vi "Previous Station Check.vi"() -> ()   [LabVIEW 2015]
uses:
  Control Button/rpt.ctl
  <vilib>/Utility/error.llb/whitespace.ctl
  <vilib>/addons/database/Connection.llb/DB Tools Open Connec (String).vi
  Galobal variable_TI.vi
  <vilib>/Utility/file.llb/Read Delimited Spreadsheet (string).vi
  Project Setup/Globle Variable/GR_Servo.vi
  <vilib>/Utility/file.llb/Write Delimited Spreadsheet (string).vi
  <vilib>/addons/database/NI_Database_API.lvlib
panel:
  out "error out 5":errorcluster
  out "array 2":string[][](array[string])
  out "error out 4":errorcluster
  out "size(s)":i32
  out "error out 3":errorcluster
  out "array":string[][](array[string])
  out "error out 2":errorcluster
  out "error out":errorcluster
  in  "stop":bool
  in  "RPT":T1
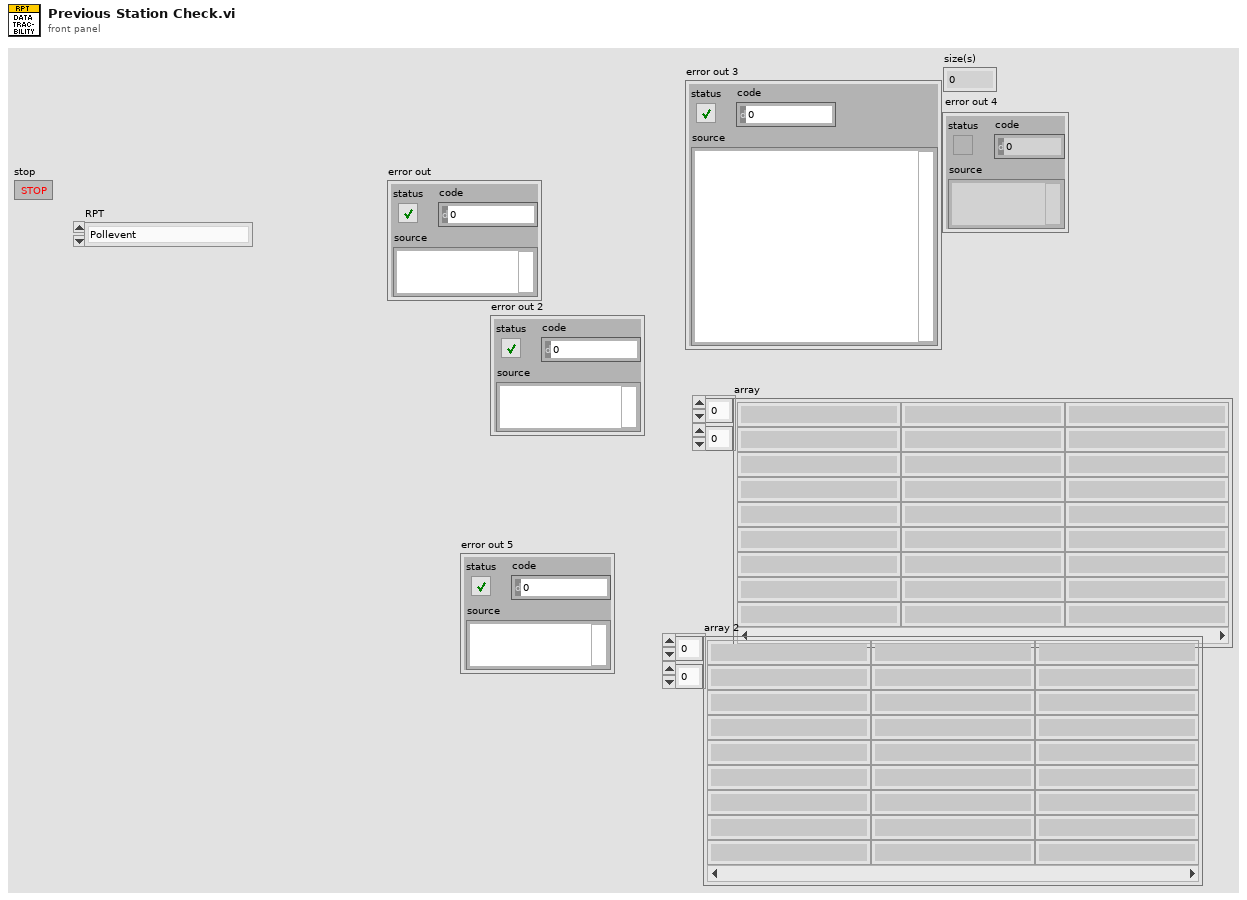
[diagram p1: front panel]
types:
  T1 = typedef "rpt.ctl" = enum16{"Pollevent", "Read", "Write", "Delete"}
  T2 = cluster{"Stn Name":string, "date":string, "time":string, "Operator id":string, "Shift":string, "Error Code":string, "Fail count":string, "Rework":string, "NA":string, "Tested":string}
  T3 = typedef "NI_Database_API.lvlib/Conn ObjectReference.ctl" = refnum<k1>
  T4 = enum16{"open", "replace", "create", "open or create", "replace or create", "replace or create with confirmation"}
  T5 = typedef "whitespace.ctl" = u16
  T6 = cluster{"Report data[0]":string, "Report data[1]":string, "Report data[2]":string, "Report data[3]":string, "Report data[4]":string, "Report data[5]":string, "Report data[6]":string, "Report data[7]":string, "Report data[8]":string, "Report data[9]":string, "Report data[10]":string, "Report data[11]":string, "Report data[12]":string, "Report data[13]":string, "Report data[14]":string, "Report data[15]":string}
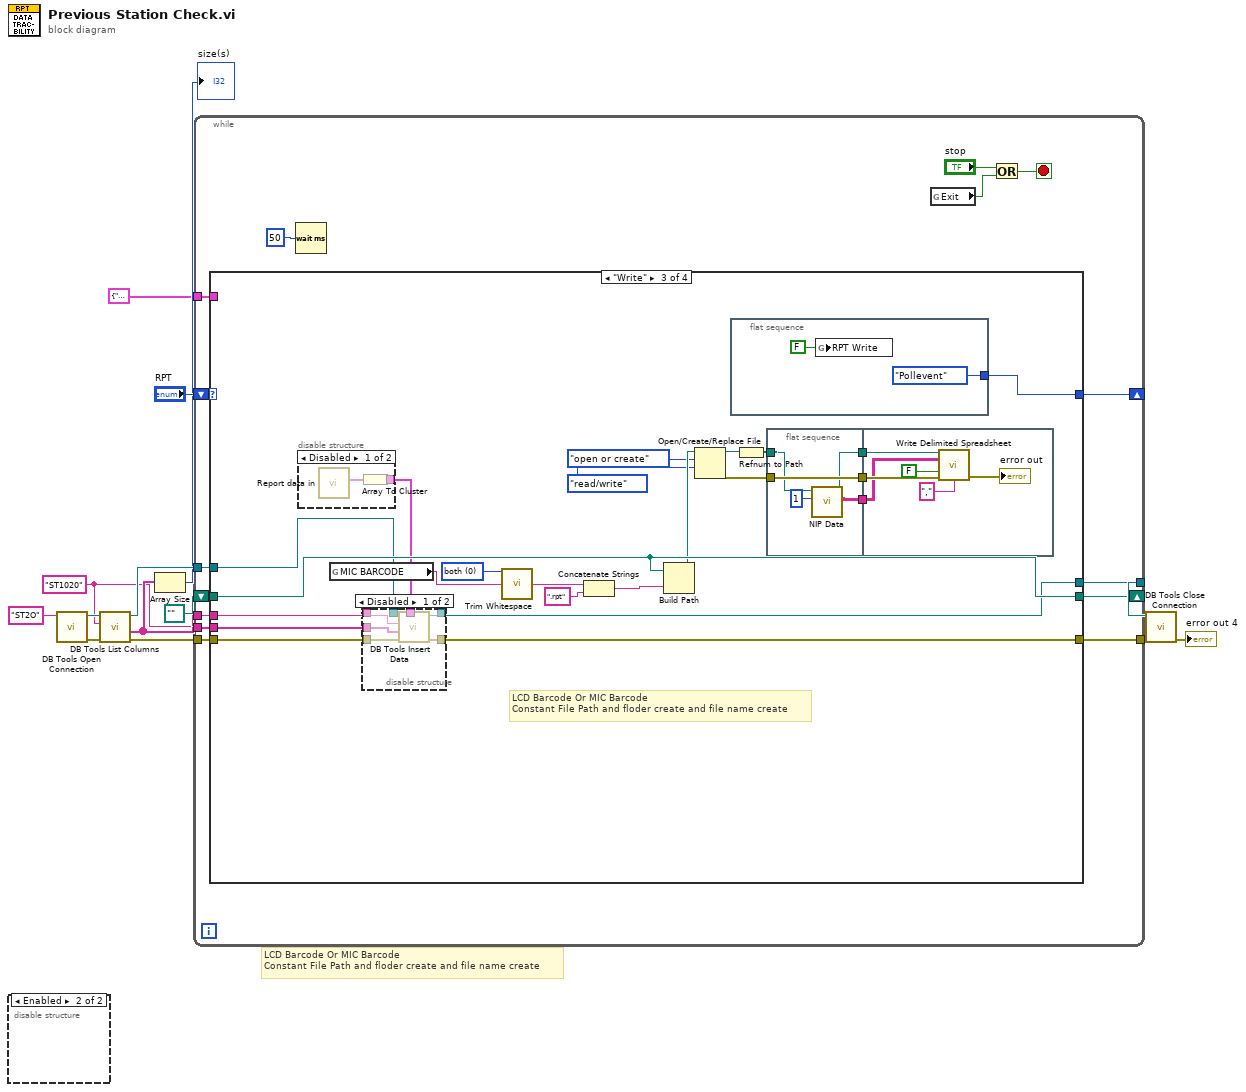
[diagram p0: block diagram]
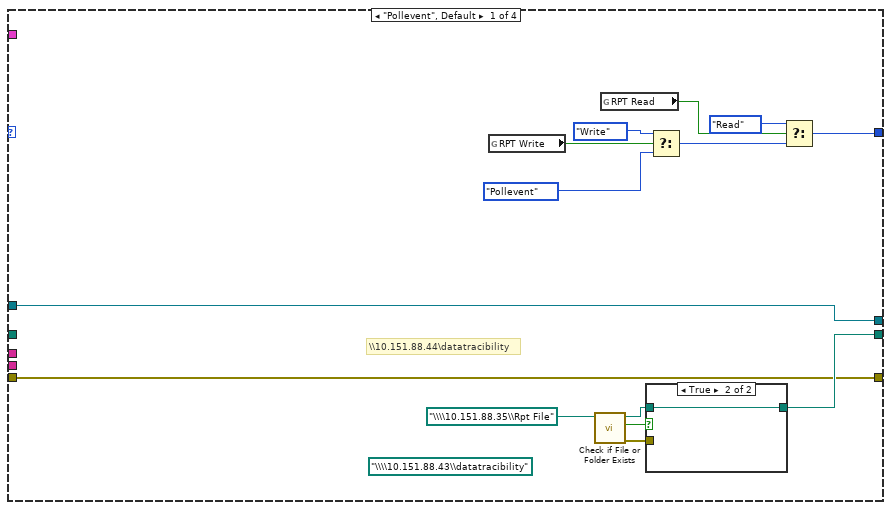
[diagram p2: hidden frame]
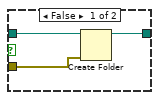
[diagram p3: hidden frame]
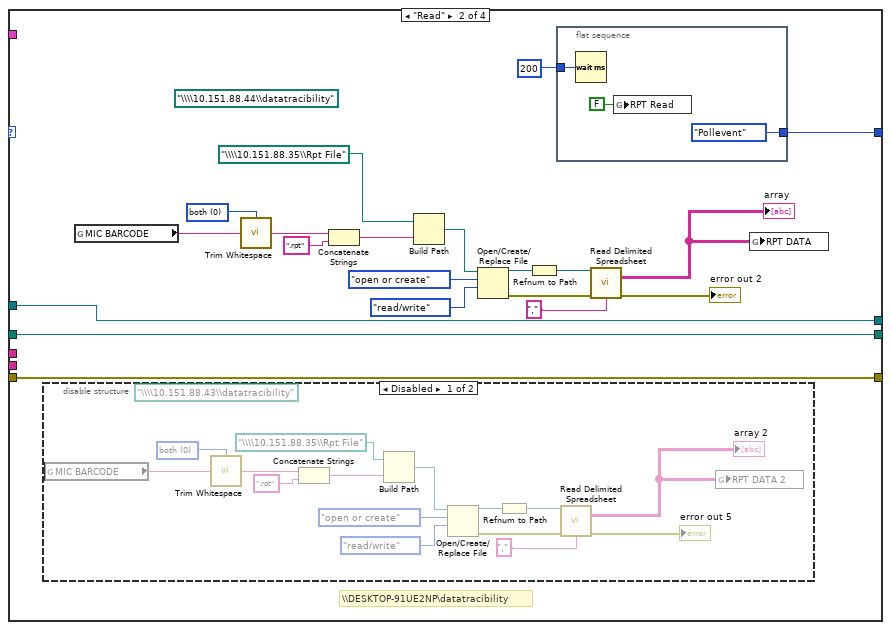
[diagram p4: hidden frame]
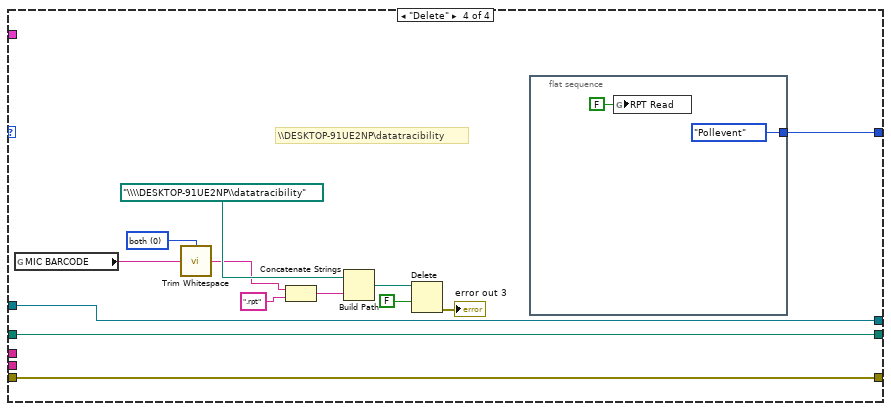
[diagram p8: hidden frame]
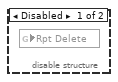
[diagram p9: hidden frame]
diagram:
  w6 = "ST1020" ("table")
  # "LCD Barcode Or MIC Barcode \nConstant File Path and floder create and file name create"
  n1 = disable-structure shown="Enabled" {
    frame Disabled {
      n2 = global read "Galobal variable_TI.vi" "Rpt Delete"() -> ()  [unwired: 1 in]
    }
    frame Enabled {
    }
  }
  n3 = call-poly <vilib>:"DB Tools Open Connection.vi"("connection information"="ST2O" ("string")) -> ("error out"=w11:errorcluster, "connection reference"=w12:T3)  [unwired: 7 in]
  n4 = call <vilib>:"DB Tools List Columns.vi"("error in (no error)"=w11, "table"=w6, "connection reference"=w12) -> ("error out"=w8:errorcluster, "columns"=w7:string[], "connection reference out"=w9:T3)  [unwired: 1 in, 1 out]
  n5 = Array Size(array=w7) -> (size(s)=→"size(s)":i32)
  n6 = while {
    shift-right: [w29] -> _
    shift-left: "RPT" -> [w28]
    shift-right: [w27] -> _
    shift-left: path "" ("created path") -> [w26]
    tunnel: w9 -> [w21]
    tunnel: w8 -> [w20]
    tunnel: w7 -> [w19]
    tunnel: w6 -> [w18]
    tunnel: [w17] -> w5
    tunnel: [w16] -> w4
    tunnel: T2 {"Stn Name"="", "date"="", "time"="", "Operator id"="", "Shift"="", "Error Code"="", "Fail count"="", "Rework"="", "NA"="", "Tested"=""} ("Write Data") -> [w15]
    stop <- w22 stop-if-true
    n7 = case shown="\"Write\"" w28 {
      tunnel: [w37 w67 w108 w143] -> w29
      tunnel: [w32 w61 w105 w140] -> w27
      tunnel: w26 -> [_ w61 w105 w140]
      tunnel: w21 -> [w31 w58 w98 w136]
      tunnel: w20 -> [w30 w57 w97 w135]
      tunnel: w19 -> [_ _ w96 _]
      tunnel: w18 -> [_ _ w95 _]
      tunnel: [w31 w58 w94 w136] -> w17
      tunnel: [w30 w57 w93 w135] -> w16
      tunnel: w15 -> [_ _ _ _]
      frame "Pollevent", Default {
        (unwired) path "\\\\10.151.88.43\\datatracibility" ("base path")
        # "\\\\10.151.88.44\\datatracibility"
        n8 = global read "Galobal variable_TI.vi" "RPT Write"() -> (w41:bool)
        n9 = call <vilib>:"Check if File or Folder Exists.vi"("path"=path "\\\\10.151.88.35\\Rpt File" ("base path")) -> ("error out"=w33:errorcluster, "file or folder exists?"=w35:bool, "dup path"=w34:path)  [unwired: 8 in]
        n10 = global read "Galobal variable_TI.vi" "RPT Read"() -> (w42:bool)
        n11 = case shown="True" w35 {
          tunnel: w34 -> [w46 w47]
          tunnel: w33 -> [w45 _]
          tunnel: [w44 w47] -> w32
          frame False {
            n12 = Create Folder(path (use dialog)=w46, error in=w45) -> (created path=w44:path)  [unwired: 1 in, 2 out]
          }
          frame True {
          }
        }
        n13 = Select(t=rpt."Write" ("RPT"), s=w41, f=rpt."Pollevent" ("RPT")) -> (s? t:f=w39:T1)
        n14 = Select(t=rpt."Read" ("RPT"), s=w42, f=w39) -> (s? t:f=w37:T1)
      }
      frame "Read" {
        (unwired) path "\\\\10.151.88.44\\datatracibility" ("base path")
        w55 = T5 0 items=["both", "start of string", "end of string"] ("location (both)")
        # "\\\\DESKTOP-91UE2NP\\datatracibility"
        n15 = disable-structure shown="Disabled" {
          frame Disabled {
            (unwired) path "\\\\10.151.88.43\\datatracibility" ("base path")
            w75 = T5 0 items=["both", "start of string", "end of string"] ("location (both)")
            n16 = global read "Galobal variable_TI.vi" "MIC BARCODE"() -> (w74:string)
            n17 = call <vilib>:"Trim Whitespace.vi"("string"=w74, "location (both)"=w75) -> ("trimmed string"=w76:string)
            n18 = Concatenate Strings(w76, ".rpt" ("string")) -> (w69:string)
            n19 = Build Path(base path=path "\\\\10.151.88.35\\Rpt File", name or relative path=w69) -> (appended path=w70:path)
            n20 = Open/Create/Replace File(file path (use dialog)=w70, operation (0:open)=T4."open or create", access (0:read/write)=enum16{"read/write", "read-only", "write-only"}."read/write") -> (refnum out=w78:refnum<file>, error out=w73:errorcluster)  [unwired: 3 in, 1 out]
            n21 = Refnum to Path(1:w78) -> (0:w79:path)
            n22 = call-poly <vilib>:"Read Delimited Spreadsheet.vi"("file path (dialog if empty)"=w79, "error in (no error)"=w73, "delimiter (\\t)"="," ("delimiter (\\t)")) -> ("all rows"=w81:string[][], "error out"=→"error out 5":errorcluster)  [unwired: 7 in, 4 out]
            "array 2" <- w81
            n23 = global write "GR_Servo.vi" "RPT DATA 2"(w81) -> ()
          }
          frame Enabled {
          }
        }
        n24 = global read "Galobal variable_TI.vi" "MIC BARCODE"() -> (w56:string)
        n25 = call <vilib>:"Trim Whitespace.vi"("string"=w56, "location (both)"=w55) -> ("trimmed string"=w54:string)
        n26 = Concatenate Strings(w54, ".rpt" ("string")) -> (w65:string)
        n27 = Build Path(base path=path "\\\\10.151.88.35\\Rpt File", name or relative path=w65) -> (appended path=w64:path)
        n28 = Open/Create/Replace File(file path (use dialog)=w64, operation (0:open)=T4."open or create", access (0:read/write)=enum16{"read/write", "read-only", "write-only"}."read/write") -> (refnum out=w52:refnum<file>, error out=w60:errorcluster)  [unwired: 3 in, 1 out]
        n29 = Refnum to Path(1:w52) -> (0:w51:path)
        n30 = flat-sequence {
          tunnel: [rpt."Pollevent" ("RPT")] -> w67
          tunnel: u32 200 ("milliseconds to wait") -> [w83]
          frame #0 {
            n31 = Wait (ms)(milliseconds to wait=w83) -> ()  [unwired: 1 out]
            n32 = global write "Galobal variable_TI.vi" "RPT Read"(FALSE ("Rpt Read")) -> ()
          }
        }
        n33 = call-poly <vilib>:"Read Delimited Spreadsheet.vi"("file path (dialog if empty)"=w51, "error in (no error)"=w60, "delimiter (\\t)"="," ("delimiter (\\t)")) -> ("all rows"=w49:string[][], "error out"=→"error out 2":errorcluster)  [unwired: 7 in, 4 out]
        "array" <- w49
        n34 = global write "GR_Servo.vi" "RPT DATA"(w49) -> ()
      }
      frame "Write" {
        w89 = T5 0 items=["both", "start of string", "end of string"] ("location (both)")
        # "LCD Barcode Or MIC Barcode \nConstant File Path and floder create and file name create"
        n35 = disable-structure shown="Disabled" {
          disable-tunnel: [w120 _] -> w92
          frame Disabled {
            n36 = call "Report data in.vi"() -> ("Report data"=w121:string[])  [unwired: 11 in]
            n37 = Array To Cluster(array=w121) -> (cluster=w120:T6)
          }
          frame Enabled {
          }
        }
        n38 = global read "Galobal variable_TI.vi" "MIC BARCODE"() -> (w91:string)
        n39 = disable-structure shown="Disabled" {
          disable-tunnel: w98 -> [w128 _]
          disable-tunnel: w97 -> [w127 _]
          disable-tunnel: w96 -> [w126 _]
          disable-tunnel: w95 -> [w125 _]
          disable-tunnel: [w124 _] -> w94
          disable-tunnel: [w123 _] -> w93
          disable-tunnel: w92 -> [w122 _]
          frame Disabled {
            n40 = call <vilib>:"DB Tools Insert Data.vi"("data"=w122, "error in (no error)"=w127, "columns"=w126, "table"=w125, "connection reference"=w128) -> ("error out"=w123:errorcluster, "connection reference out"=w124:T3)  [unwired: 5 in]
          }
          frame Enabled {
          }
        }
        n41 = call <vilib>:"Trim Whitespace.vi"("string"=w91, "location (both)"=w89) -> ("trimmed string"=w90:string)
        n42 = Concatenate Strings(w90, ".rpt" ("string")) -> (w106:string)
        n43 = Build Path(base path=w105, name or relative path=w106) -> (appended path=w104:path)
        n44 = Open/Create/Replace File(file path (use dialog)=w104, operation (0:open)=T4."open or create", access (0:read/write)=enum16{"read/write", "read-only", "write-only"}."read/write") -> (refnum out=w101:refnum<file>, error out=w99:errorcluster)  [unwired: 3 in, 1 out]
        n45 = flat-sequence {
          tunnel: [rpt."Pollevent" ("RPT")] -> w108
          frame #0 {
            n46 = global write "Galobal variable_TI.vi" "RPT Write"(FALSE ("Rpt Read")) -> ()
          }
        }
        n47 = Refnum to Path(1:w101) -> (0:w100:path)
        n48 = flat-sequence {
          tunnel: w99 -> [w113]
          tunnel: w100 -> [w112]
          tunnel: [w110] -> w88
          tunnel: [w113] -> w87
          tunnel: [w109] -> w86
          tunnel: w88 -> [w119]
          tunnel: w87 -> [w118]
          tunnel: w86 -> [w114]
          frame #0 {
            n49 = call "NIP Data.vi"("index (row)"=1, "file path (dialog if empty)"=w112) -> ("Data"=w109:string[][], "file path (dialog if empty) 2"=w110:path)  [unwired: 8 in]
          }
          frame #1 {
            n50 = call-poly <vilib>:"Write Delimited Spreadsheet.vi"("file path (dialog if empty)"=w119, "2D data"=w114, "append to file? (F)"=FALSE, "error in (no error)"=w118, "delimiter (\\t)"="," ("delimiter (\\t)")) -> ("error out"=→"error out":errorcluster)  [unwired: 9 in, 1 out]
          }
        }
      }
      frame "Delete" {
        w133 = T5 0 items=["both", "start of string", "end of string"] ("location (both)")
        # "\\\\DESKTOP-91UE2NP\\datatracibility"
        n51 = global read "Galobal variable_TI.vi" "MIC BARCODE"() -> (w132:string)
        n52 = call <vilib>:"Trim Whitespace.vi"("string"=w132, "location (both)"=w133) -> ("trimmed string"=w131:string)
        n53 = Concatenate Strings(w131, ".rpt" ("string")) -> (w141:string)
        n54 = Build Path(base path=path "\\\\DESKTOP-91UE2NP\\datatracibility", name or relative path=w141) -> (appended path=w139:path)
        n55 = Delete(path (use dialog)=w139, confirm (F)=FALSE) -> (error out=→"error out 3":errorcluster)  [unwired: 3 in, 2 out]
        n56 = flat-sequence {
          tunnel: [rpt."Pollevent" ("RPT")] -> w143
          frame #0 {
            n57 = global write "Galobal variable_TI.vi" "RPT Read"(FALSE ("Rpt Read")) -> ()
          }
        }
      }
    }
    n58 = Wait (ms)(milliseconds to wait=u32 50) -> ()  [unwired: 1 out]
    n59 = global read "Galobal variable_TI.vi" "Exit"() -> (w24:bool)
    n60 = Or(x="stop", y=w24) -> (x .or. y?=w22:bool)
  }
  n61 = call <vilib>:"DB Tools Close Connection.vi"("error in (no error)"=w4, "connection reference"=w5) -> ("error out"=→"error out 4":errorcluster)  [unwired: 5 in]
